vi "GetHourList.vi"() -> (3 "Hour List":string[](array[string]))   [LabVIEW 2017, in "UI_TimeSelector.xctl"]
uses:
  UI_TimeSelector/UI_TimeSelector.xctl
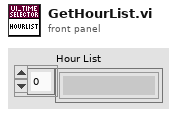
[diagram p1: front panel]
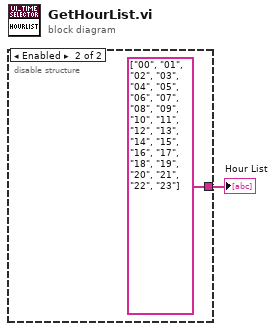
[diagram p0: block diagram]
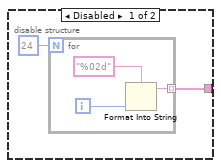
[diagram p2: hidden frame]
diagram:
  n1 = disable-structure shown="Enabled" {
    disable-tunnel: [w3 string[] ["00", "01", "02", "03", "04", "05", "06", "07", "08", "09", "10", "11", "12", "13", "14", "15", "16", "17", "18", "19", "20", "21", "22", "23"] ("Hour List")] -> w1
    frame Disabled {
      n2 = for {
        N: 24 -> [_]
        tunnel: [w5] -> w3 mode=indexing
        i -> [w6]
        n3 = Format Into String(format string="%02d", w6) -> (resulting string=w5:string)  [unwired: 2 in, 1 out]
      }
    }
    frame Enabled {
    }
  }
  "Hour List" <- w1
